vi "main_load_environtment.vi"(3 "Hydrolysis spec":refnum<vi>, 4 "Flow":refnum<vi>, 5 "Methane spec":refnum<vi>, 6 "Starttime":refnum<vi>, 7 "Env. Dir":refnum<vi>, 8 "Env. Ready?":refnum<vi>, 9 "Environtment Tree":refnum<vi>, 10 "Load Env":refnum<vi>, 11 "Running?":refnum<vi>) -> ()   [LabVIEW 2019]
uses:
  <vilib>/Utility/sysdir.llb/System Directory Type.ctl
  lib/libSimulationControl/libSimulationControl.lvlib
panel:
  # "*******************************************************************\nBiogas Plant Control\n\nAuthor: Paul Zügel\nGCSC-Frankfurt am Main 2020\n\n*******************************************************************"
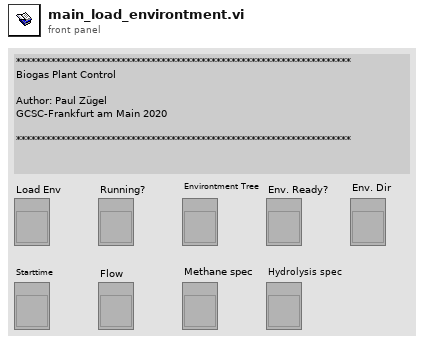
[diagram p1: front panel]
types:
  T1 = enum8{"Enabled", "Disabled", "Disabled and Grayed Out"}
  T2 = typedef "System Directory Type.ctl" = i32
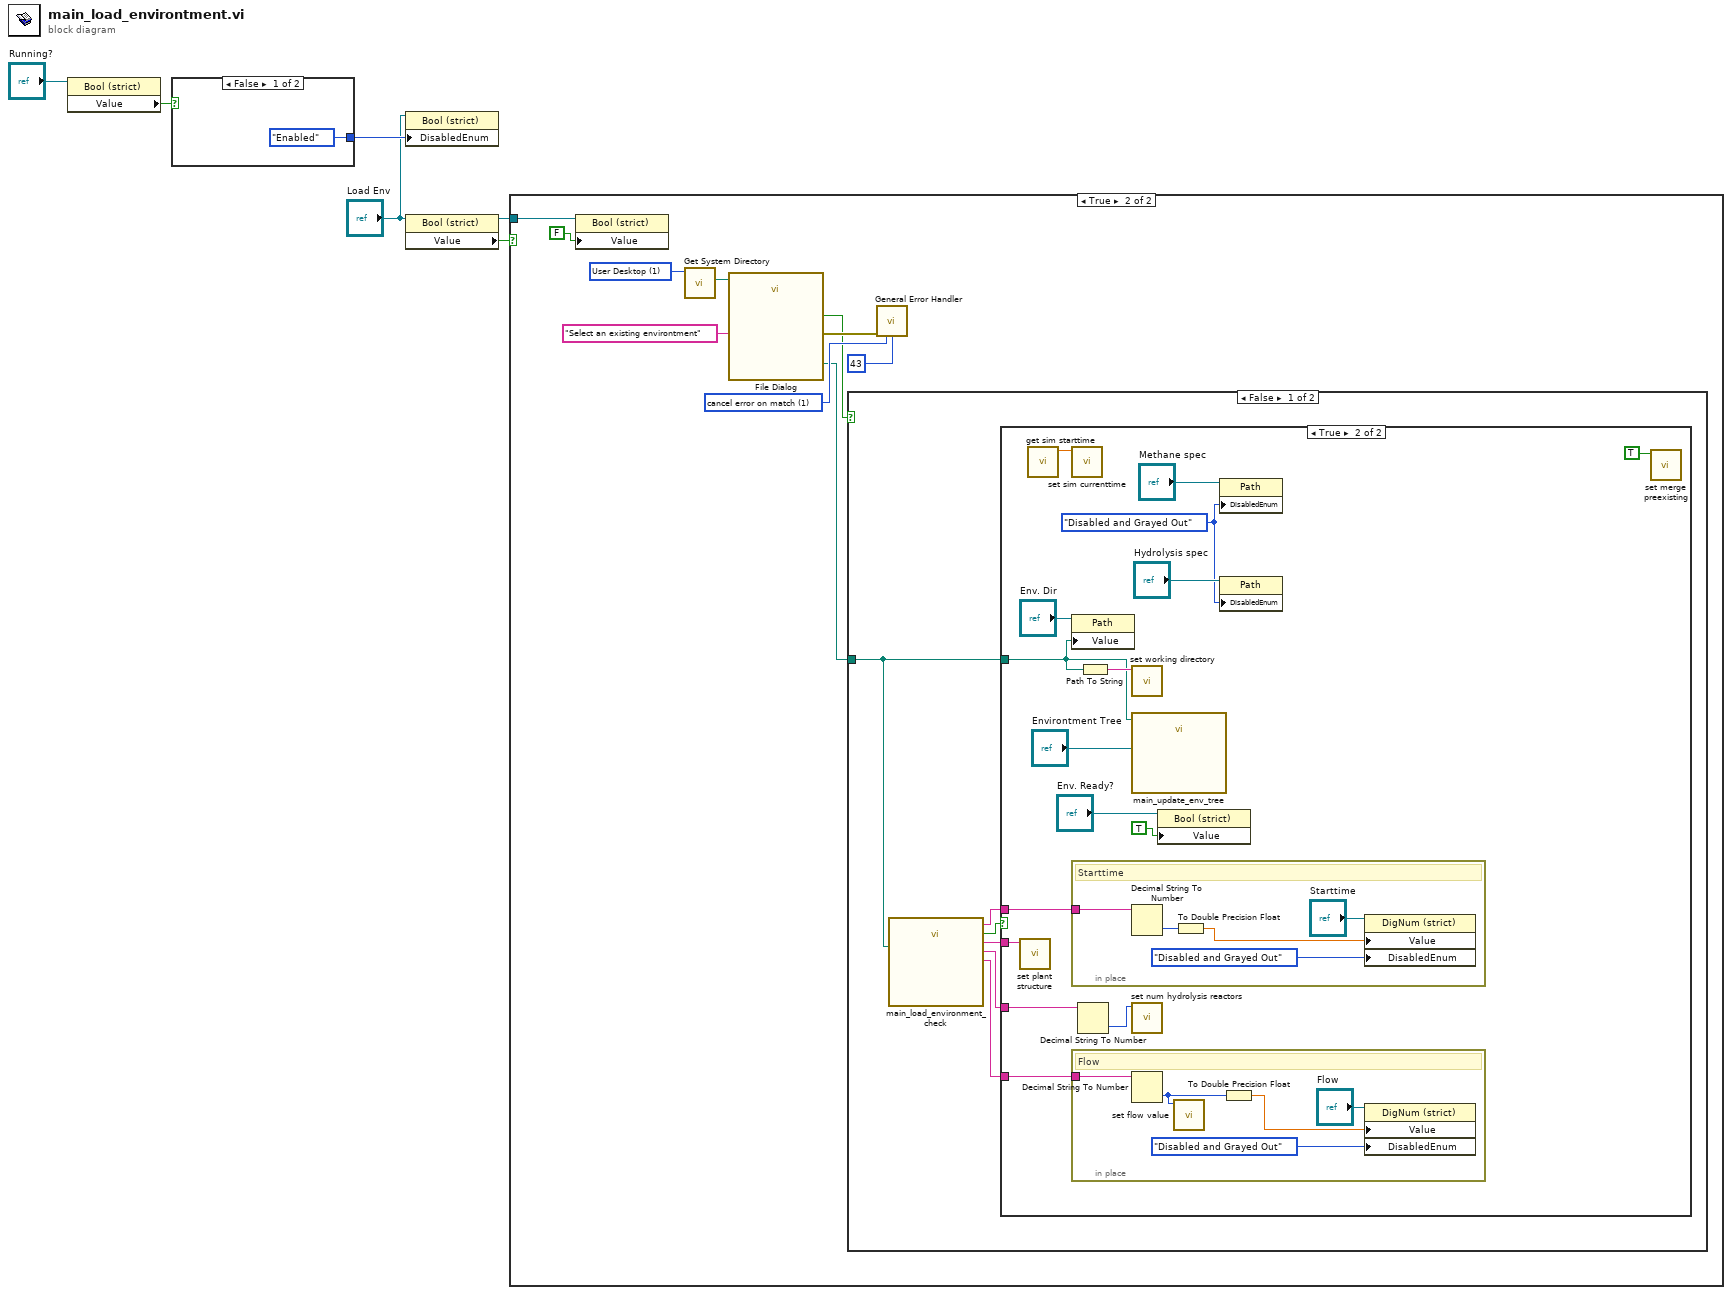
[diagram p0: block diagram]
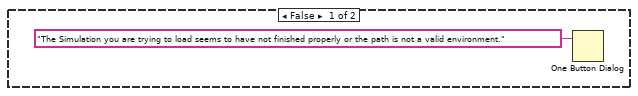
[diagram p3: hidden frame]
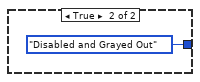
[diagram p5: hidden frame]
diagram:
  n1 = property class="Bool (strict)"(reference="Running?") -> ("Value"=w5:bool)  [unwired: 1 in, 2 out]
  n2 = case shown="False" w5 {
    tunnel: [T1."Enabled" ("Disabled") T1."Disabled and Grayed Out" ("Disabled")] -> w4
    frame False {
    }
    frame True {
    }
  }
  n3 = property class="Bool (strict)"(reference="Load Env", "DisabledEnum"=w4) -> ()  [unwired: 1 in, 2 out]
  n4 = property class="Bool (strict)"(reference="Load Env") -> (reference out=w1:refnum<vi>, "Value"=w2:bool)  [unwired: 1 in, 1 out]
  n5 = case shown="True" w2 {
    tunnel: w1 -> [_ w18]
    frame False {
    }
    frame True {
      w14 = T2 1 items=["User Home"=0, "User Desktop"=1, "User Documents"=2, "User Application Data"=3, "User Preferences"=4, "User Temporary"=5, "Public Documents"=6, "Public Application Data"=7, "Public Preferences"=8, "Public Cache"=13, "System Core Libraries"=9, "System Installed Libraries"=10, "Application Files"=11, "Boot Volume Root"=12] ("system directory type")
      w13 = 1 items=["no exception", "cancel error on match", "set error on match"] ("[exception action] (none:0)")
      n6 = property class="Bool (strict)"(reference=w18, "Value"=FALSE) -> ()  [unwired: 1 in, 2 out]
      n7 = call <vilib>:"Get System Directory.vi"("system directory type"=w14) -> ("system directory"=w16:path)  [unwired: 10 in]
      n8 = call "File Dialog"("start path"=w16, "prompt"="Select an existing environtment") -> ("selected path"=w9:path, "cancelled"=w10:bool, "error out"=w15:errorcluster)  [unwired: 10 in, 1 out]
      n9 = case shown="False" w10 {
        tunnel: w9 -> [w24 _]
        frame False {
          n10 = call "main_load_environment_check.vi"("New working Dir"=w24) -> ("Num_Hydro"=w20:string, "Structure"=w21:string, "Valid?"=w23:bool, "Endtime"=w22:string, "FlowVal"=w19:string)  [unwired: 6 in]
          n11 = case shown="True" w23 {
            tunnel: w24 -> [_ w31]
            tunnel: w22 -> [_ w36]
            tunnel: w21 -> [_ w35]
            tunnel: w20 -> [_ w34]
            tunnel: w19 -> [_ w29]
            frame False {
              n12 = One Button Dialog(message="The Simulation you are trying to load seems to have not finished properly or the path is not a valid environment.") -> ()  [unwired: 1 in, 1 out]
            }
            frame True {
              w26 = T1."Disabled and Grayed Out" ("Disabled")
              n13 = call "set plant structure.vi"("structure"=w35) -> ()  [unwired: 10 in, 1 out]
              n14 = call "get sim starttime.vi"() -> ("sim_starttime"=w32:dbl)  [unwired: 10 in, 1 out]
              n15 = call "set sim currenttime.vi"("time"=w32) -> ()  [unwired: 10 in, 1 out]
              n16 = property class="Path"(reference="Env. Dir", "Value"=w31) -> ()  [unwired: 1 in, 2 out]
              n17 = in-place {
                in-place-border: w36 -> [w44]
                # "Starttime"
                n18 = Decimal String To Number(string=w44) -> (number=w42:i32)  [unwired: 2 in, 1 out]
                n19 = To Double Precision Float(number=w42) -> (double precision float=w43:dbl)
                n20 = property class="DigNum (strict)"(reference="Starttime", "Value"=w43, "DisabledEnum"=T1."Disabled and Grayed Out" ("Disabled")) -> ()  [unwired: 1 in, 2 out]
              }
              n21 = in-place {
                in-place-border: w29 -> [w48]
                # "Flow"
                n22 = Decimal String To Number(string=w48) -> (number=w47:i32)  [unwired: 2 in, 1 out]
                n23 = call "set flow value.vi"("val"=w47) -> ()  [unwired: 10 in, 1 out]
                n24 = To Double Precision Float(number=w47) -> (double precision float=w51:dbl)
                n25 = property class="DigNum (strict)"(reference="Flow", "Value"=w51, "DisabledEnum"=T1."Disabled and Grayed Out" ("Disabled")) -> ()  [unwired: 1 in, 2 out]
              }
              n26 = Decimal String To Number(string=w34) -> (number=w33:i32)  [unwired: 2 in, 1 out]
              n27 = Path To String(path=w31) -> (string=w41:string)
              n28 = call "set working directory.vi"("dir"=w41) -> ()  [unwired: 10 in, 1 out]
              n29 = call "main_update_env_tree.vi"("Env. Tree"="Environtment Tree", "Env_path"=w31) -> ()  [unwired: 10 in]
              n30 = call "set num hydrolysis reactors.vi"("num"=w33) -> ()  [unwired: 10 in, 1 out]
              n31 = property class="Bool (strict)"(reference="Env. Ready?", "Value"=TRUE) -> ()  [unwired: 1 in, 2 out]
              n32 = property class="Path"(reference="Methane spec", "DisabledEnum"=w26) -> ()  [unwired: 1 in, 2 out]
              n33 = property class="Path"(reference="Hydrolysis spec", "DisabledEnum"=w26) -> ()  [unwired: 1 in, 2 out]
              n34 = call "set merge preexisting.vi"("merge"=TRUE) -> ()  [unwired: 10 in, 1 out]
            }
          }
        }
        frame True {
        }
      }
      n35 = call <vilib>:"General Error Handler.vi"("error in (no error)"=w15, "[exception action] (none:0)"=w13, "[exception code]"=43) -> ()  [unwired: 8 in, 5 out]
    }
  }
